vi "ActionVIOnCompile.vi"(8 "error in":errorcluster, 11 "Device Item Ref in":T1 format="%.0x") -> (0 "error out":errorcluster)   [LabVIEW 2026, in "Nominal Core Streaming System Explorer.lvlib"]
uses:
  Nominal Core Streaming System Explorer.lvlib
  <vilib>/NI VeriStand/Custom Device API/Custom Device Item Ref.ctl
  Shared/Compiled.Settings.ctl
  Shared/compiled stream data.ctl
  Shared/stream configuration mode.ctl
  Shared/time convert type.ctl
  <vilib>/NI VeriStand/Custom Device API/Get Item Property (U16).vi
  <vilib>/NI VeriStand/Custom Device API/Set Item Property (Variant).vi
  <vilib>/NI VeriStand/Custom Device API/Custom Device API.lvlib
  <vilib>/NI/NIVS Inline Async API/_Data Access System Explorer/Data Access System Explorer.lvlib
  Shared/Nominal Core Streaming Shared.lvlib
  <vilib>/Utility/SystemLogging/NI_SystemLogging.lvlib
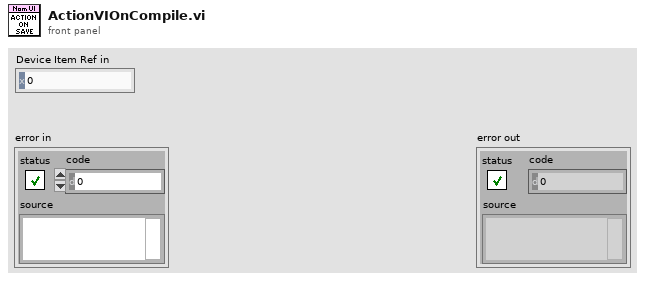
[diagram p1: front panel]
types:
  T1 = typedef "Custom Device API.lvlib/Custom Device Item Ref.ctl" = u64
  T2 = typedef "Nominal Core Streaming Shared.lvlib/Compiled.Settings.ctl" = cluster{"Name":string, "Async Init Timeout":u16, "stream":T3}
  T3 = typedef "Nominal Core Streaming Shared.lvlib/compiled stream data.ctl" = cluster{"stream name":string, "Base URL":string, "api key":string, "identifier selection":T4, "asset ID":string, "dataset name":string, "dataset ID":string, "associated channels":cluster{"Name":string, "Path":string}[], "fallback avro path":path, "time source":T5, "buffer size":u32}
  T4 = typedef "Nominal Core Streaming Shared.lvlib/stream configuration mode.ctl" = enum16{"Asset Identifier and Dataset Name", "Dataset Identifier"}
  T5 = typedef "Nominal Core Streaming Shared.lvlib/time convert type.ctl" = enum16{"to timestamp", "relative seconds"}
  T6 = typedef "Custom Device API.lvlib/Custom Device Item Info.ctl" = cluster{"Name":string, "Is Channel":bool, "GUID":string, "Is Waveform":bool}
  T7 = cluster{"Name":string, "Type":enum16{"Output/Write", "Input/Read", "Input/ReadWrite"}, "VS Refs":T1[]}[]
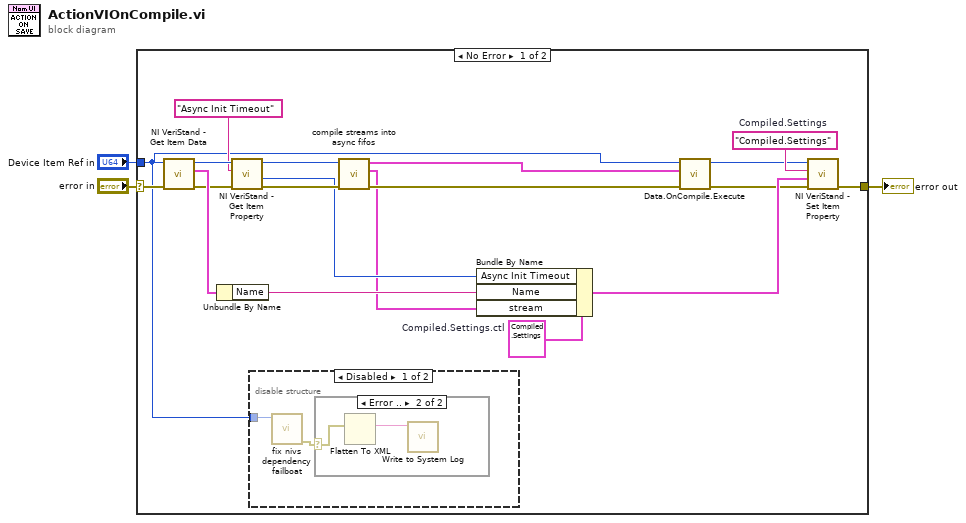
[diagram p0: block diagram]
diagram:
  n1 = case shown="No Error" "error in" {
    selector: "error in" -> [w19 w27]
    tunnel: [w20 w27] -> w2
    tunnel: "Device Item Ref in" -> [w5 _]
    frame No Error {
      w13 = T2 {"Name"="", "Async Init Timeout"=0, "stream"={"stream name"="", "Base URL"="https://api.gov.nominal.io/api/", "api key"="", "identifier selection"=enum."Asset Identifier and Dataset Name", "asset ID"="", "dataset name"="", "dataset ID"="", "associated channels"=[], "fallback avro path"=path "", "time source"=enum."to timestamp", "buffer size"=0}}  # Compiled.Settings.ctl
      w22 = "Compiled.Settings"  # Compiled.Settings
      n2 = call <vilib>:"NI VeriStand - Get Item Data.vi"("error in (no error)"=w19, "Item Ref in"=w5) -> ("error out"=w12:errorcluster, "Item Info"=w18:T6, "Item Ref out"=w10:T1)  [unwired: 6 in, 1 out]
      n3 = Unbundle By Name(w18) -> ("Name"=w17:string)
      n4 = call-poly <vilib>:"NI VeriStand - Get Item Property.vi"("error in (no error)"=w12, "Property Name"="Async Init Timeout", "Item Ref in"=w10) -> ("error out"=w11:errorcluster, "Value"=w7:u16, "Item Ref out"=w9:T1)  [unwired: 5 in, 1 out]
      n5 = disable-structure shown="Disabled" {
        disable-tunnel: w5 -> [w24 _]
        frame Disabled {
          n6 = call "fix nivs dependency failboat.vi"("Device Item Ref in"=w24) -> ("error out"=w23:errorcluster)  [unwired: 10 in]
          n7 = case shown="Error .." w23 {
            selector: w23 -> [_ w25]
            frame #0 {
            }
            frame #1 {
              n8 = Flatten To XML(6:w25) -> (2:w26:string)
              n9 = call <vilib>:"Write to System Log.vi"("message"=w26) -> ()  [unwired: 10 in, 1 out]
            }
          }
        }
        frame Enabled {
        }
      }
      n10 = call "compile streams into async fifos.vi"("error in"=w11, "CD in"=w9) -> ("error out"=w16:errorcluster, "compiled stream data"=w6:T3, "fifo groups"=w4:T7)  [unwired: 7 in]
      n11 = Bundle By Name(cluster=w13, "Async Init Timeout"=w7, "Name"=w17, "stream"=w6) -> (w21:T2)
      n12 = call <vilib>:"Data.OnCompile.Execute.vi"("error in"=w16, "VS Ref Groups"=w4, "Custom Device Ref"=w5) -> ("error out"=w15:errorcluster, "Custom Device Ref"=w14:T1)  [unwired: 7 in]
      n13 = call-poly <vilib>:"NI VeriStand - Set Item Property.vi"("error in (no error)"=w15, "Value"=w21, "Property Name"=w22, "Item Ref in"=w14) -> ("error out"=w20:errorcluster)  [unwired: 5 in, 2 out]
    }
    frame Error {
    }
  }
  "error out" <- w2
